vi "Simple File Download.vi"() -> ()   [LabVIEW 2018]
doc: "Uploads, or sends, a relatively small local file to a remote SSH server. This is similar to the SCP command line utility when transferring, or copying, a local file to a remote destination. If performance is poor or memory is limited on the local machine, then it could be because the file is relatively large and this implementation is not very efficient for relatively large files."
uses:
  Toolkit/API/File Info/File Info.lvclass/File Info.ctl
  Toolkit/API/SSH/SSH.lvclass/SSH.ctl
  Toolkit/API/SSH/Utility/Read Shared Library.vi
  Toolkit/API/Session/Support/Password Authentication.vi
  Toolkit/API/File Info/Support/Create from Session.vi
  Toolkit/API/Channel/Support/Create from SCP Receive.vi
  Toolkit/Support/Check Status.vi
  Toolkit/API/File Info/Support/Destroy to Channel.vi
  Toolkit/API/Channel/Support/Destroy to Session.vi
  Toolkit/API/SSH/SSH.lvclass
  Toolkit/API/Session/Session.lvclass
  Toolkit/API/Channel/Channel.lvclass
  Toolkit/API/File Info/File Info.lvclass
panel:
  in  "Remote File":string
  in  "Local File":path
  in  "Remote SSH Server":string
  in  "Password":string
  in  "Username":string
  # "Overview: Demonstrates transferring, or downloading, a remote file from a SSH server, similar to the SCP command line utility\nInstructions:\n1. Enter the IP address or host name of the remote SSH server. This can be a CompactRIO (cRIO) running the National Instruments Linux Real-Time (NI Linux RT) operating system with the Enable Secure Shell Server (sshd) checkbox checked. \n2. Enter a username. If using a cRIO with a default configuration, then the username is \"admin\".\n3. Enter a password for the username. If using a cRIO with a default configuration, then the password is blank (empty).\n4. Select a file on the local computer to transfer/upload to the remote SSH server.\n5. Enter a path and/or filename for the uploaded file on the remote SSH server. Typically, this is a POSIX/UNIX file path with a backslash, \"/\", use to separate directories and the default directory is the remote user's home directory, i.e. \"/home/admin\" on a default configured cRIO.\n6. Run this VI."
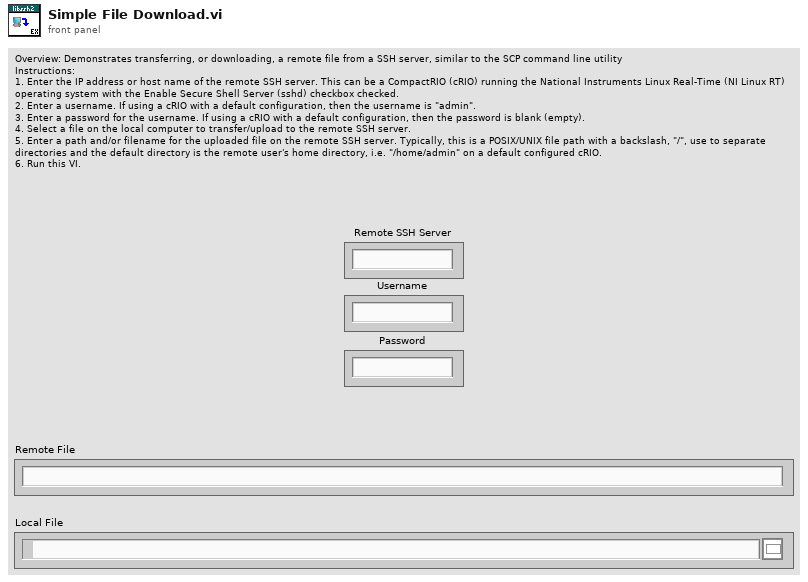
[diagram p1: front panel]
types:
  T1 = enum16{"open", "replace", "create", "open or create", "replace or create", "replace or create with confirmation"}
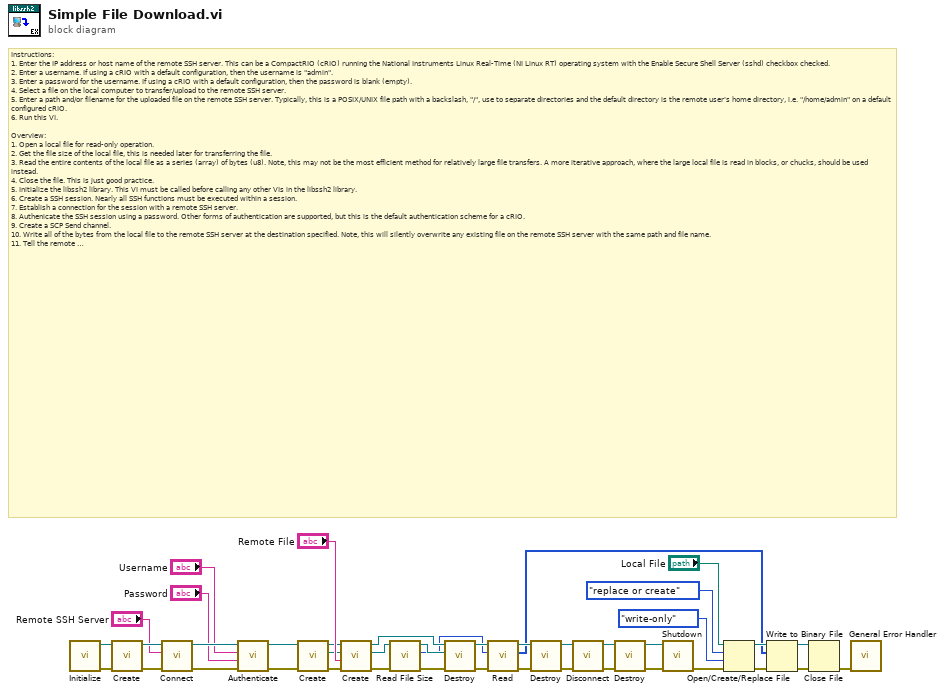
[diagram p0: block diagram]
diagram:
  # "Instructions:\n1. Enter the IP address or host name of the remote SSH server. This can be a CompactRIO (cRIO) running the National Instruments Linux Real-Time (NI Linux RT) operating system with the Enable Secure Shell Server (sshd) checkbox checked. \n2. Enter a username. If using a cRIO with a default configuration, then the username is \"admin\".\n3. Enter a password for the username. If using a cRIO with a default configuration, then the password is blank (empty).\n4. Select a file on the local computer to transfer/upload to the remote SSH server.\n5. Enter a path and/or filename for the uploaded file on the remote SSH server. Typically, this is a POSIX/UNIX file path with a backslash, \"/\", use to separate directories and the default directory is the remote user's home directory, i.e. \"/home/admin\" on a default configured cRIO.\n6. Run this VI.\n\nOverview:\n1. Open a local file for read-only operation.\n2. Get the file size of the local file, this is needed later for transferring the file.\n3. Read the entire contents of the local file as a series (array) of bytes (u8). Note, this may not be the most efficient method for relatively large file transfers. A more iterative approach, where the large local file is read in blocks, or chucks, should be used instead.\n4. Close the file. This is just good practice.\n5. Initialize the libssh2 library. This VI must be called before calling any other VIs in the libssh2 library.\n6. Create a SSH session. Nearly all SSH functions must be executed within a session.\n7. Establish a connection for the session with a remote SSH server.\n8. Authenicate the SSH session using a password. Other forms of authentication are supported, but this is the default authentication scheme for a cRIO. \n9. Create a SCP Send channel.\n10. Write all of the bytes from the local file to the remote SSH server at the destination specified. Note, this will silently overwrite any existing file on the remote SSH server with the same path and file name.\n11. Tell the remote SSH server that all of the bytes from the local file have been sent to it and no more bytes will be sent. Also, wait for the remote SSH server to acknowledge that the file transfer is complete. This is not strictly required, but it is good practice.\n12. Close the SCP Send channel. Again, not strictly required, but it is good practice.\n13. Destroy the SCP Send channel. Since the \"Create\" VI is used, the complementary \"Destroy\" VI must be used to free resources within the libssh2 library.\n14. Disconnect from the remote SSH server.\n15. Destroy the session to free resources within the libssh2 library.\n16. Shutdown the libssh2 library. This VI must be last VI called for the libssh2 library. No other libssh2 VIs should be called once this VI is executed.\n17. Provide some error handling and reporting. Libssh2 errors will be in the -8100 range."
  n1 = call "Initialize.vi"() -> ("Error Out"=w27:errorcluster, "SSH"=w26:refnum<class "SSH.lvclass">)  [unwired: 10 in]
  n2 = call "Create.vi"("Error In"=w27, "SSH"=w26) -> ("Error Out"=w40:errorcluster, "Sesssion"=w41:refnum<class "Session.lvclass">)  [unwired: 8 in]
  n3 = call "Connect.vi"("Error In"=w40, "Address"="Remote SSH Server", "Session In"=w41) -> ("Error Out"=w38:errorcluster, "Sesssion Out"=w39:refnum<class "Session.lvclass">)  [unwired: 7 in]
  n4 = call-poly "Authenticate.vi"("Error In"=w38, "Password"="Password", "Username"="Username", "Session In"=w39) -> ("Error Out"=w22:errorcluster, "Sesssion Out"=w25:refnum<class "Session.lvclass">)  [unwired: 6 in]
  n5 = call-poly "Create.vi"("Error In"=w22, "Session In"=w25) -> ("Error Out"=w21:errorcluster, "File Info"=w23:refnum<class "File Info.lvclass">, "Session Out"=w24:refnum<class "Session.lvclass">)  [unwired: 7 in]
  n6 = call-poly "Create.vi"("Error In"=w21, "Remote Source Path"="Remote File", "File Info In"=w23, "Session"=w24) -> ("Error Out"=w18:errorcluster, "File Info Out"=w19:refnum<class "File Info.lvclass">, "Channel"=w20:refnum<class "Channel.lvclass">)  [unwired: 5 in]
  n7 = call "Read File Size.vi"("Error In"=w18, "File Info In"=w19) -> ("Error Out"=w16:errorcluster, "File Size"=w13:u64, "File Info Out"=w17:refnum<class "File Info.lvclass">)  [unwired: 7 in]
  n8 = call-poly "Destroy.vi"("Error In"=w16, "File Info"=w17, "Channel In"=w20) -> ("Error Out"=w14:errorcluster, "Channel Out"=w15:refnum<class "Channel.lvclass">)  [unwired: 7 in]
  n9 = call "Read.vi"("Error In"=w14, "Max Data Length"=w13, "Channel In"=w15) -> ("Error Out"=w11:errorcluster, "Data"=w4:u8[], "Channel Out"=w12:refnum<class "Channel.lvclass">)  [unwired: 5 in, 1 out]
  n10 = call-poly "Destroy.vi"("Error In"=w11, "Channel"=w12) -> ("Error Out"=w33:errorcluster, "Session"=w34:refnum<class "Session.lvclass">)  [unwired: 8 in]
  n11 = call "Disconnect.vi"("Error In"=w33, "Session In"=w34) -> ("Error Out"=w31:errorcluster, "Sesssion Out"=w32:refnum<class "Session.lvclass">)  [unwired: 8 in]
  n12 = call "Destroy.vi"("Error In"=w31, "Session"=w32) -> ("Error Out"=w29:errorcluster, "SSH"=w30:refnum<class "SSH.lvclass">)  [unwired: 8 in]
  n13 = call "Shutdown.vi"("Error In"=w29, "SSH"=w30) -> ("Error Out"=w10:errorcluster)  [unwired: 9 in]
  n14 = Open/Create/Replace File(file path (use dialog)="Local File", error in=w10, operation (0:open)=T1."replace or create", access (0:read/write)=enum16{"read/write", "read-only", "write-only"}."write-only") -> (refnum out=w6:refnum<file>, error out=w5:errorcluster)  [unwired: 2 in, 1 out]
  n15 = Write to Binary File(file (use dialog)=w6, data=w4, error in=w5) -> (refnum out=w3:refnum<file>, error out=w2:errorcluster)  [unwired: 3 in, 1 out]
  n16 = Close File(refnum=w3, error in=w2) -> (error out=w1:errorcluster)  [unwired: 1 out]
  n17 = call <vilib>:"General Error Handler.vi"("error in (no error)"=w1) -> ()  [unwired: 10 in, 5 out]
